vi "my_min_function.vi"(6 "first image height":dbl, 7 "first cut height":dbl, 8 "Error In":errorcluster, 10 "image height":dbl[](array[numeric]) format="%#_13g", 11 "cut height":dbl[](array[numeric]) format="%#_13g") -> (0 "Error out":errorcluster, 2 "min value":dbl)   [LabVIEW 2018]
uses:
  Controls/FGV Actions.ctl
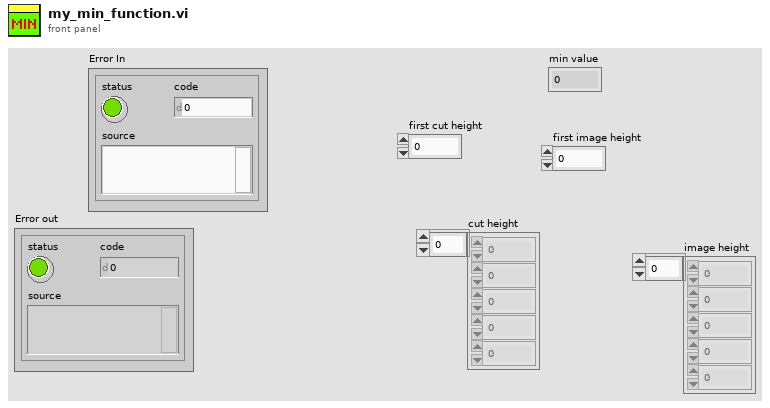
[diagram p1: front panel]
types:
  T1 = typedef "FGV Actions.ctl" = enum16{"Init", "Set", "Get", "Clear"}
  T2 = typedef "System Parameters.ctl" = cluster{"Optical Parameters":T3, "Vibratome":T4, "Table Stages":T6, "Imaging Parameter":T9, "Galvo HW Parameters":cluster{"Analog Out Channel":tag, "Min Voltage":dbl, "Max Voltage":dbl, "Pixel Clock Source":tag, "Sample Rate":dbl, "Line Clock Out Ch":tag, "2P ready check":tag}, "Alazar parameters":T11, "Mosaic Paramter":cluster{"X Axis":cluster{"Start [mm]":dbl, "Steps [pts]":dbl, "End [mm]":dbl}, "Y Axis":cluster{"Start [mm]":dbl, "Steps [pts]":dbl, "End [mm]":dbl}, "Scan Pattern":enum16{"Uni-directional", "Bi-Directional", "Spiral Out", "Spiral In"}, "Overlap Options":cluster{"Overlap Type":enum16{"No Overlap", "X Only", "Y Only", "X and Y"}, "Percent Overlap":u8, "Justify":enum16{"Start", "Center", "End"}}}, "Manual Controls":T18, "Z stage setting":T21, "Attenuator":T22}
  T3 = typedef "Optical Parameters.ctl" = cluster{"Obj. Focal Length [mm]":dbl, "Scan Lens EFL[mm]":dbl, "Tube Lens EFL[mm]":dbl, "Galvo V Range (+/-)":dbl, "Galvo Max Half Angle [Deg]":dbl, "Max Galvo Range[%]":dbl}
  T4 = typedef "Vibratome Parameters.ctl" = cluster{"Pre Cut Dwell [s]":dbl, "Blade Frequency [RPM]":u16, "Slice Speed [mm/s]":dbl, "Post Cut Dwell [s]":dbl, "Ramp Time [s]":dbl, "Start X [mm]":dbl, "Start Y [mm]":dbl, "Slice Length [mm]":dbl, "Slice Axis":enum16{"X Axis", "Y Axis", "Z Axis"}, "Controller VISA Ref":refnum<visa-resource-name>, "Blade Frequency [Hz]":u16, "Analog Out Channel":tag, "Pixel Clock Source":tag, "Vib version":T5}
  T5 = typedef "vibratome.ctl" = enum16{"Vibratome1", "Vibratome3"}
  T6 = typedef "Translation Stage Parameters.ctl" = cluster{"X Stage":T7, "Y Stage":T7, "Z Stage":T7, "Attenuator":T7}
  T7 = typedef "Translation Stage Cluster.ctl" = cluster{"Position":dbl, "Is.Enabled?":bool, "Is.Connected?":bool, "Device SN":string, "AccelerationMaximum":dbl, "VelocityMaximum":dbl, "Acceleration":dbl, "Velocity":dbl, "waitTimeout (ms)":i32, "Model":T8, "Is.Homed?":bool, "MOVE":bool}
  T8 = typedef "Translation Stage Types.ctl" = enum16{"None", "Thorlabs LTS", "Thorlabs MLJ"}
  T9 = typedef "Imaging Parameters.ctl" = cluster{"Raster Scan Direction":T10, "Pixel Dwell Time [Clock Cycles]":u16, "Flyback Time [Clock Cycles]":u16, "XY Center [um]":cluster{"X":dbl, "Y":dbl}, "Pixel Step Size [um] X":dbl, "XY Image Size":enum16{"32 x 32", "64 x 64", "128 x 128", "256 x 256", "512 x 512", "1024 x 1024", "2048 x 2048"}, "Custom":bool, "Custom Size":cluster{"X":u16, "Y":u16}, "Line Averages":u8, "Pixel Step Size [um] Y":dbl}
  T10 = typedef "Scan Direction.ctl" = enum16{"Uni Directional", "Bi Directional", "None"}
  T11 = typedef "Alazar parameters.ctl" = cluster{"Trigger Settings":cluster{"General Trigger Settings":T12, "Trigger Engine 1":T13, "Trigger Engine 2":T13}, "Device ID":T14, "Ch A Input Control":T15, "Ch B Input Control":T15, "Acq Settings":T16, "Capture Clock":T17}
  T12 = typedef "General Trigger Settings.ctl" = cluster{"Trigger Operation":u32, "Coupling ID":u32, "Range ID":u32, "Delay":u32, "Timeout Ticks":u32, "Mode":u32, "Parameter":u32}
  T13 = typedef "Trigger Engine Controls.ctl" = cluster{"Trigger Engine":u32, "Source":u32, "Slope":u32, "Level":u32}
  T14 = typedef "Alazar Device ID.ctl" = cluster{"System ID":u32, "Board ID":u32}
  T15 = typedef "Channel Input Controls.ctl" = cluster{"Channel":u8, "Coupling":u32, "Range":u32, "Impedance":u32}
  T16 = typedef "Alazar Acquisition Settings.ctl" = cluster{"Record Length":u32, "Offset":u32, "Records Per Buffer":u32, "Records Count (Records/Acq)":u32, "Window Type":u32, "Footer":u32, "Samples per record":u32, "Output Format":u32}
  T17 = typedef "Clock Controls.ctl" = cluster{"Sample Rate":u32, "Decimation":u32, "Source":u32, "Edge":u32}
  T18 = typedef "Manual Controls.ctl" = cluster{"Data Path":path, "Save parameters":T19, "Center Galvos":bool, "Acquisition mode":T20, "PSOCT Channel":u32, "Save data?":bool, "AIP rotation angle":dbl, "Pause acquisition?":bool, "Outgoing Mail Server (SMTP)":string, "Email":string, "Password":string, "Carrier 1":enum16{"T-Mobile", "AT&T", "Verizon", "Sprint"}, "phone number 1":string, "Subject":string, "Message":string, "Carrier 2":enum16{"T-Mobile", "AT&T", "Verizon", "Sprint"}, "phone number 2":string, "Check boundary?":bool, "Threshold":sgl, "ret downsample?":bool}
  T19 = typedef "FFT parameters.ctl" = cluster{"start pixel":i32, "#pixels to save":i32}
  T20 = typedef "FFT mode.ctl" = enum16{"ThorOCT B line", "ThorOCT Spectral", "ThorOCT FFT", "Alazar B line", "Alazar FFT", "GPU FFT", "Alazar Spectral", "Simulation", "auto adjust focus", "Save all"}
  T21 = typedef "Vibratome Param.ctl" = cluster{"first cut height(mm)":dbl, "slice thickness[um]":dbl[], "#repetitions":u16, "image thickness(um)":dbl[], "#cycles per repetition":u16, "First image height(mm)":dbl, "Block?":bool[], "Z0":dbl, "fixed Z0?":bool}
  T22 = typedef "attenuator.ctl" = cluster{"Power after Objective (recalibrate every 6 month)":dbl[]}
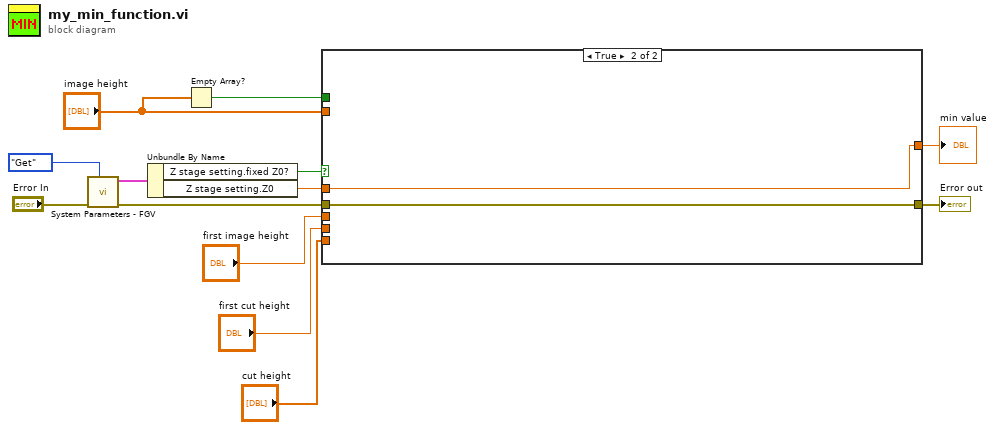
[diagram p0: block diagram]
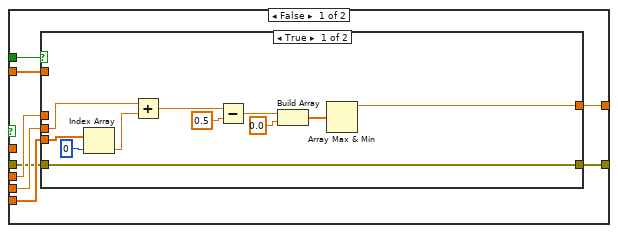
[diagram p2: hidden frame]
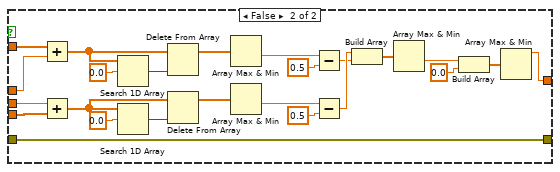
[diagram p3: hidden frame]
diagram:
  n1 = call "System Parameters - FGV.vi"("Actions"=FGV_Actions."Get", "Error In"="Error In") -> ("Error Out"=w2:errorcluster, "System Parameters [Out]"=w6:T2)  [unwired: 8 in]
  n2 = Unbundle By Name(w6) -> ("Z stage setting.fixed Z0?"=w5:bool, "Z stage setting.Z0"=w4:dbl)
  n3 = Empty Array?(array="image height") -> (empty?=w10:bool)
  n4 = case shown="True" w5 {
    tunnel: [w21 w58] -> w13
    tunnel: "cut height" -> [w20 _]
    tunnel: "image height" -> [w19 _]
    tunnel: w10 -> [w18 _]
    tunnel: "first cut height" -> [w17 _]
    tunnel: "first image height" -> [w16 _]
    tunnel: w4 -> [_ w58]
    tunnel: w2 -> [w15 w57]
    tunnel: [w14 w57] -> w1
    frame False {
      n5 = case shown="True" w18 {
        tunnel: [w26 w40] -> w21
        tunnel: w20 -> [w32 w39]
        tunnel: w19 -> [_ w36]
        tunnel: w17 -> [w25 w35]
        tunnel: w16 -> [_ w34]
        tunnel: w15 -> [w22 w33]
        tunnel: [w22 w33] -> w14
        frame True {
          n6 = Index Array(array=w32, index=0) -> (element=w24:dbl)
          n7 = Add(x=w25, y=w24) -> (x+y=w23:dbl)
          n8 = Subtract(x=w23, y=0.5) -> (x-y=w27:dbl)
          n9 = Build Array(w27, 0.0 ("element")) -> (w29:dbl[])
          n10 = Array Max & Min(array=w29) -> (max value=w26:dbl)  [unwired: 3 out]
        }
        frame False {
          n11 = Add(x=w36, y=w34) -> (x+y=w37:dbl[])
          n12 = Add(x=w35, y=w39) -> (x+y=w38:dbl[])
          n13 = Search 1D Array(1D array=w37, element=0.0) -> (index of element=w45:i32)  [unwired: 1 in]
          n14 = Search 1D Array(1D array=w38, element=0.0) -> (index of element=w48:i32)  [unwired: 1 in]
          n15 = Delete From Array(array=w37, index=w45) -> (array with subset deleted=w44:dbl[])  [unwired: 1 in, 1 out]
          n16 = Delete From Array(array=w38, index=w48) -> (array with subset deleted=w47:dbl[])  [unwired: 1 in, 1 out]
          n17 = Array Max & Min(array=w44) -> (min value=w50:dbl)  [unwired: 3 out]
          n18 = Array Max & Min(array=w47) -> (min value=w51:dbl)  [unwired: 3 out]
          n19 = Subtract(x=w50, y=0.5) -> (x-y=w52:dbl)
          n20 = Subtract(x=w51, y=0.5) -> (x-y=w53:dbl)
          n21 = Build Array(w53, w52) -> (w56:dbl[])
          n22 = Array Max & Min(array=w56) -> (min value=w42:dbl)  [unwired: 3 out]
          n23 = Build Array(w42, 0.0 ("element")) -> (w43:dbl[])
          n24 = Array Max & Min(array=w43) -> (max value=w40:dbl)  [unwired: 3 out]
        }
      }
    }
    frame True {
    }
  }
  "min value" <- w13
  "Error out" <- w1
